vi "expParametersConfig.vi"(8 "Error IN":errorcluster caption="constante d'erreur") -> (0 "Error OUT":errorcluster caption="constante d'erreur", 1 "expParamsIsOK":bool, 3 "expConfig":T1={"colorParameters"={"giver"="", "acceptor"=[]}, "recordDataInTDMS?"=TRUE, "PID_mode"=enum."rampe"})   [LabVIEW 2020]
uses:
  defTypeConfigs/expConfig.ctl
panel:
  in  "OK":bool
  # "EXPERIENCE PARAMETERS"
  # "COLORS PARAMETERS CHOICES\nRECORD DATA IN TDMS FILE ?\nPID MODE (consigne continu ou variable)"
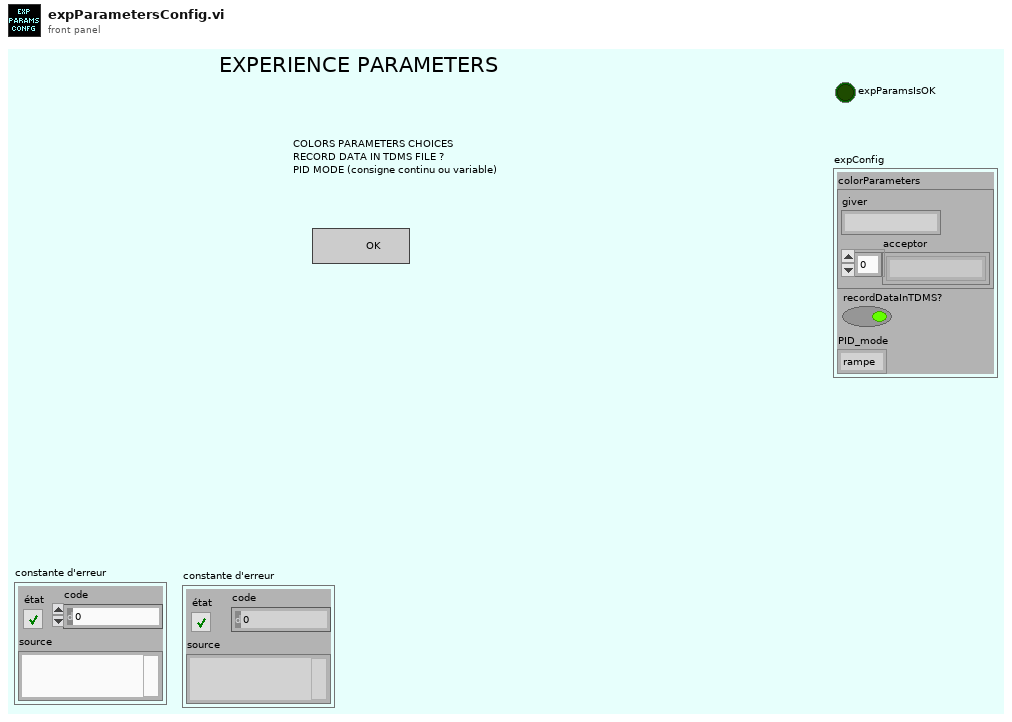
[diagram p1: front panel]
types:
  T1 = typedef "expConfig.ctl" = cluster{"colorParameters":cluster{"giver":string, "acceptor":string[]}, "recordDataInTDMS?":bool, "PID_mode":enum16{"rampe", "triangle", "sinus", "carré", "continu"}}
  T2 = enum16{"rampe", "triangle", "sinus", "carré", "continu"}
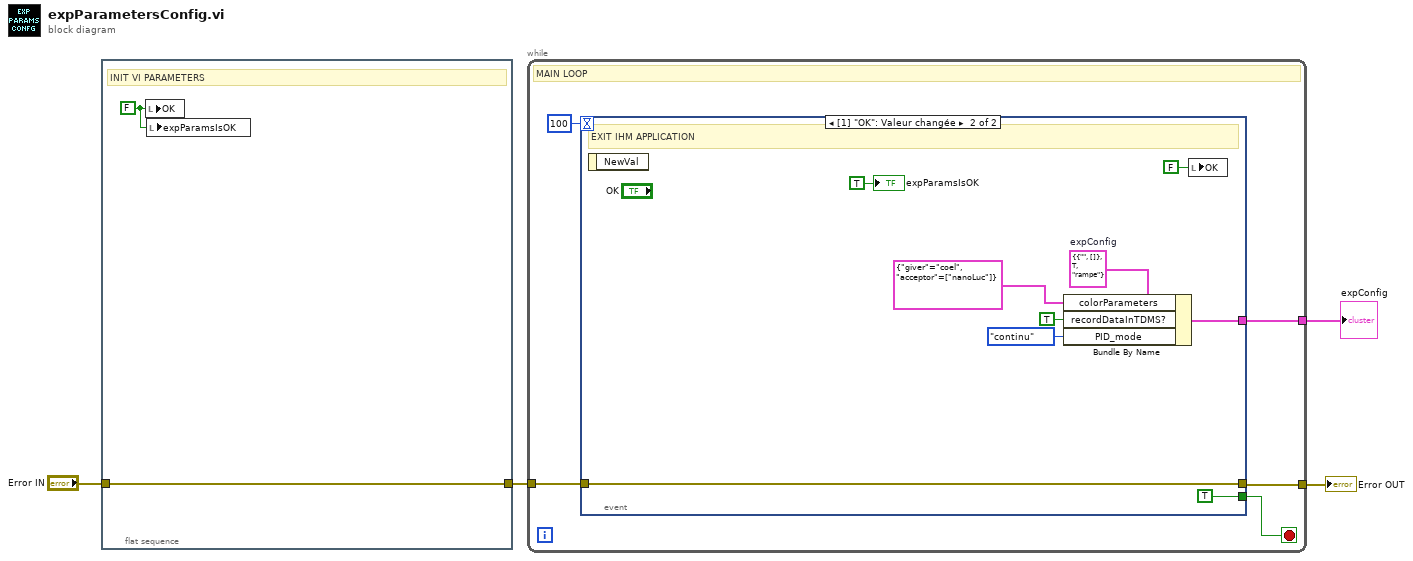
[diagram p0: block diagram]
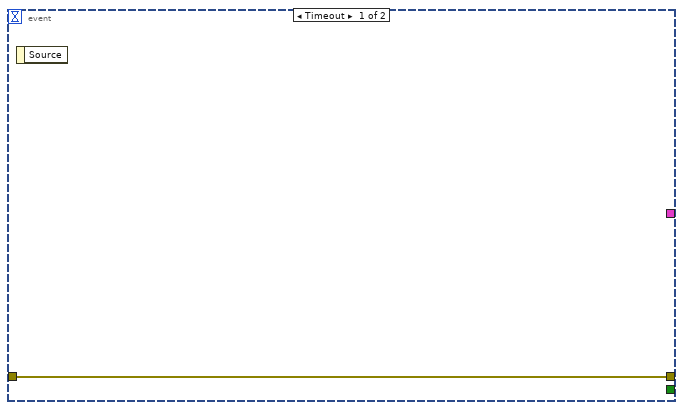
[diagram p2: hidden frame]
diagram:
  n1 = flat-sequence {
    tunnel: "Error IN" -> [w6]
    tunnel: [w6] -> w3
    frame #0 {
      w5 = FALSE ("Exit")
      # "INIT VI PARAMETERS"
      n2 = local write "OK"(w5) -> ()
      n3 = local write "expParamsIsOK"(w5) -> ()
    }
  }
  n4 = while {
    tunnel: w3 -> [w10]
    tunnel: [w9] -> w2
    tunnel: [w7] -> w1
    stop <- w8 stop-if-true
    # "MAIN LOOP"
    n5 = event shown="[1] \"OK\": Valeur changée" {
      selector: _ -> [_ _]
      dyn-events: _ -> [_ _]
      timeout: 100 -> [_ _]
      tunnel: w10 -> [w12 w20]
      tunnel: [w12 w20] -> w9
      tunnel: [_ TRUE] -> w8
      tunnel: [_ w17] -> w7
      event Timeout {
        n6 = event-data() -> ()  [unwired: 1 in, 1 out]
      }
      event "OK": Value Change {
        w16 = T1 {"colorParameters"={"giver"="", "acceptor"=[]}, "recordDataInTDMS?"=TRUE, "PID_mode"=enum."rampe"}  # expConfig
        # "EXIT IHM APPLICATION"
        n7 = event-data() -> ()  [unwired: 1 in, 1 out]
        n8 = Bundle By Name(cluster=w16, "colorParameters"=cluster{"giver":string, "acceptor":string[]} {"giver"="coel", "acceptor"=["nanoLuc"]}, "recordDataInTDMS?"=TRUE, "PID_mode"=T2."continu") -> (w17:T1)
        n9 = local write "OK"(FALSE ("Exit")) -> ()
        "expParamsIsOK" <- TRUE ("expParamsIsOK")
      }
    }
  }
  "Error OUT" <- w2
  "expConfig" <- w1
